vi "OAT Orbit Arbitrary Probe Angle Compensation.vi"(7 "select methods":bool, 8 "error in (no error)":errorcluster, 9 "probe angle":cluster{"X (red)":u32, "Y (blue)":u32}(knob)={"X (red)"=0, "Y (blue)"=90}, 11 "XY plot data in":cluster{dbl[], dbl[]}[](array[cluster]) {"?" format="%.2f"; "?" format="%.2f"}) -> (0 "error out":errorcluster, 1 "probe angle out":cluster{"X (red)":dbl, "Y (blue)":dbl}, 3 "XY plot data out":cluster{dbl[], dbl[]}[](array[cluster]) {"?" format="%.2f"; "?" format="%.2f"})   [LabVIEW 2017]
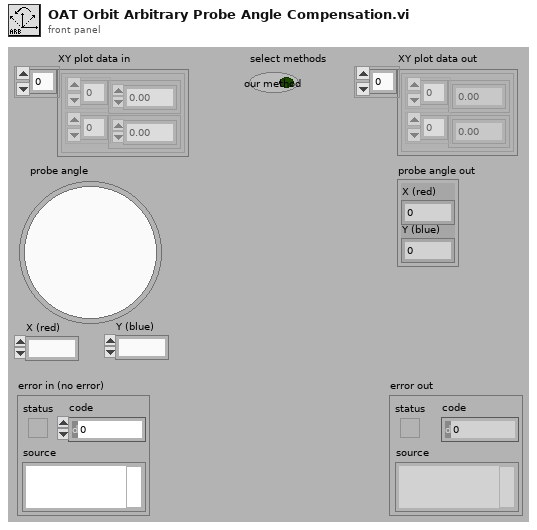
[diagram p1: front panel]
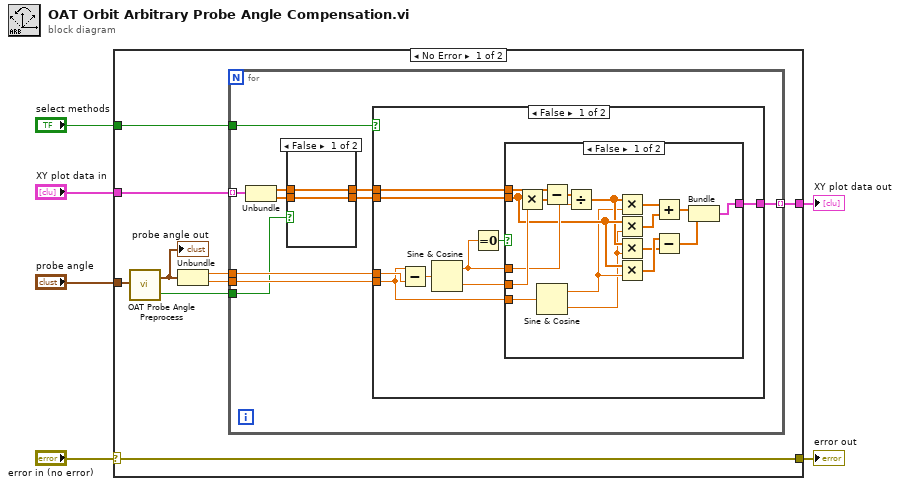
[diagram p0: block diagram]
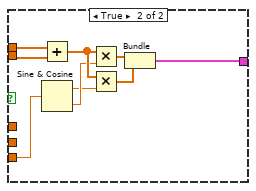
[diagram p3: hidden frame]
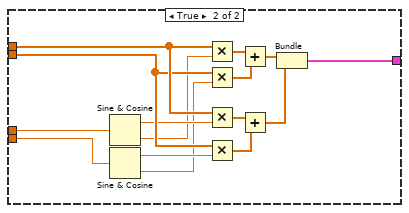
[diagram p4: hidden frame]
diagram:
  n1 = case shown="No Error" "error in (no error)" {
    selector: "error in (no error)" -> [w7 w81]
    tunnel: "XY plot data in" -> [w15 w80]
    tunnel: "select methods" -> [w14 _]
    tunnel: [w13 w80] -> w4
    tunnel: "probe angle" -> [w12 _]
    tunnel: [w7 w81] -> w1
    frame No Error {
      n2 = call <vilib>:"OAT Probe Angle Preprocess.vi"("probe angle"=w12) -> ("switch x y axis"=w8:bool, "probe angle out"=w11:cluster{"X (red)":dbl, "Y (blue)":dbl})  [unwired: 1 in]
      "probe angle out" <- w11
      n3 = Unbundle(w11) -> ("X (red)"=w10:dbl, "Y (blue)"=w9:dbl)
      n4 = for {
        tunnel: w15 -> [w23] mode=indexing
        tunnel: w14 -> [w25]
        tunnel: [w24] -> w13 mode=indexing
        tunnel: w10 -> [w22]
        tunnel: w9 -> [w21]
        tunnel: w8 -> [w20]
        n5 = Unbundle(w23) -> (w19:dbl[], w18:dbl[])
        n6 = case shown="False" w20 {
          tunnel: w19 -> [w27 w29]
          tunnel: w18 -> [w26 w28]
          tunnel: [w26 w29] -> w17
          tunnel: [w27 w28] -> w16
          frame False {
          }
          frame True {
          }
        }
        n7 = case shown="False" w25 {
          tunnel: [w37 w73] -> w24
          tunnel: w16 -> [w36 w72]
          tunnel: w17 -> [w35 w71]
          tunnel: w22 -> [w38 w70]
          tunnel: w21 -> [w30 w67]
          frame False {
            n8 = Subtract(x=w30, y=w38) -> (x-y=w33:dbl)
            n9 = Sine & Cosine(0:w33) -> (1:w32:dbl, 2:w31:dbl)
            n10 = Equal To 0?(x=w32) -> (x = 0?=w34:bool)
            n11 = case shown="False" w34 {
              tunnel: w31 -> [w55 _]
              tunnel: w32 -> [w53 _]
              tunnel: w30 -> [w45 w58]
              tunnel: [w46 w64] -> w37
              tunnel: w36 -> [w43 w63]
              tunnel: w35 -> [w48 w62]
              frame False {
                n12 = Multiply(x=w48, y=w55) -> (x*y=w52:dbl[])
                n13 = Sine & Cosine(0:w45) -> (1:w40:dbl, 2:w39:dbl)
                n14 = Subtract(x=w43, y=w52) -> (x-y=w54:dbl[])
                n15 = Divide(x=w54, y=w53) -> (x/y=w44:dbl[])
                n16 = Multiply(x=w44, y=w40) -> (x*y=w51:dbl[])
                n17 = Multiply(x=w48, y=w39) -> (x*y=w50:dbl[])
                n18 = Multiply(x=w44, y=w39) -> (x*y=w41:dbl[])
                n19 = Multiply(x=w48, y=w40) -> (x*y=w42:dbl[])
                n20 = Add(x=w51, y=w50) -> (x+y=w49:dbl[])
                n21 = Subtract(x=w42, y=w41) -> (x-y=w47:dbl[])
                n22 = Bundle(w49, w47) -> (w46:cluster{dbl[], dbl[]})  [unwired: 1 in]
              }
              frame True {
                n23 = Add(x=w63, y=w62) -> (x+y=w61:dbl[])
                n24 = Sine & Cosine(0:w58) -> (1:w56:dbl, 2:w57:dbl)
                n25 = Multiply(x=w61, y=w57) -> (x*y=w60:dbl[])
                n26 = Multiply(x=w61, y=w56) -> (x*y=w59:dbl[])
                n27 = Bundle(w60, w59) -> (w64:cluster{dbl[], dbl[]})  [unwired: 1 in]
              }
            }
          }
          frame True {
            n28 = Sine & Cosine(0:w70) -> (1:w69:dbl, 2:w68:dbl)
            n29 = Sine & Cosine(0:w67) -> (1:w66:dbl, 2:w65:dbl)
            n30 = Multiply(x=w72, y=w68) -> (x*y=w79:dbl[])
            n31 = Multiply(x=w71, y=w65) -> (x*y=w78:dbl[])
            n32 = Multiply(x=w72, y=w69) -> (x*y=w77:dbl[])
            n33 = Multiply(x=w71, y=w66) -> (x*y=w76:dbl[])
            n34 = Add(x=w79, y=w78) -> (x+y=w75:dbl[])
            n35 = Add(x=w77, y=w76) -> (x+y=w74:dbl[])
            n36 = Bundle(w75, w74) -> (w73:cluster{dbl[], dbl[]})  [unwired: 1 in]
          }
        }
      }
    }
    frame Error {
    }
  }
  "XY plot data out" <- w4
  "error out" <- w1
